vi "Overlays_test.vi"() -> ()   [LabVIEW 2018]
panel:
  out "Waveform Chart":cluster{dbl, dbl}(graph)
  in  "Stop":bool
  in  "Image Display":T1(plugin-control)
  out "size(s)":i32[](array[numeric])
  in  "Overlay Object":path=path "D:/Users_Data/Dmitriy_T/Documents/Tracker/TestVI's/Overlay_Object.png"
  in  "Overlay Bgr":path=path "D:/Users_Data/Dmitriy_T/Documents/Tracker/TestVI's/Overlay_Bgr.png"
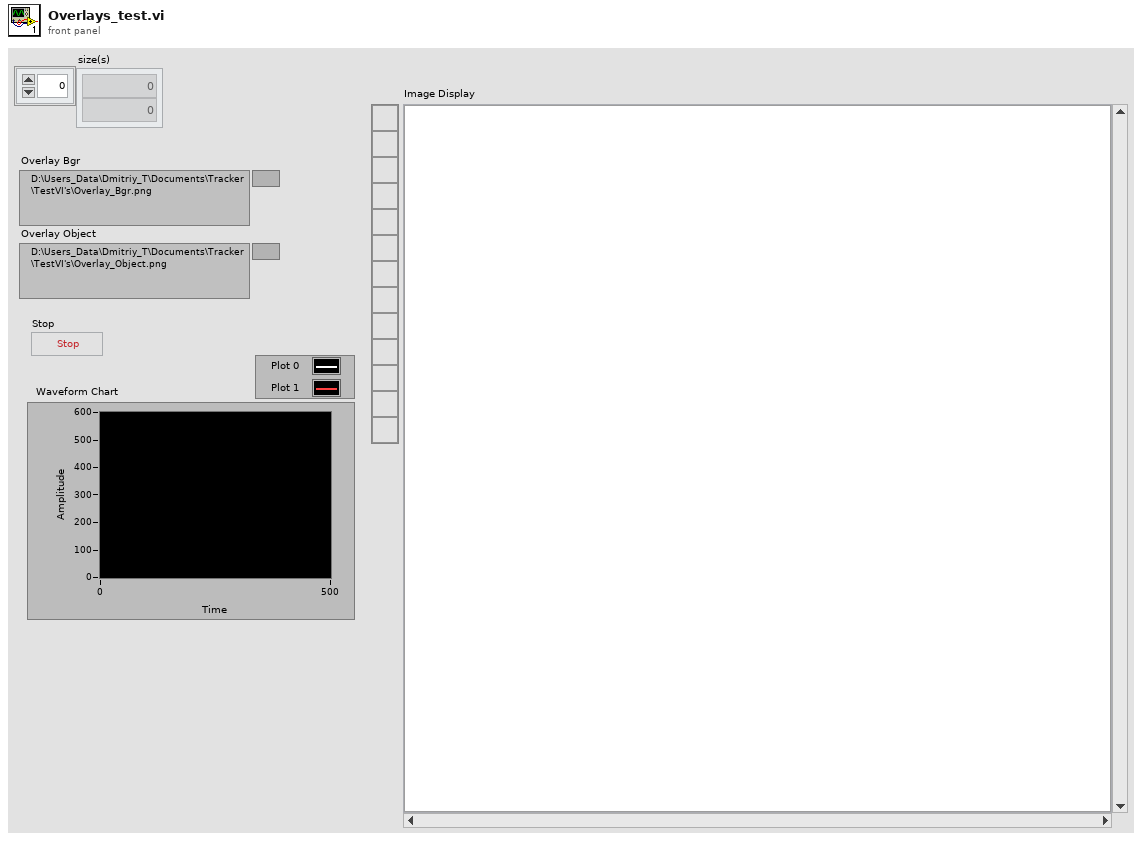
[diagram p1: front panel]
types:
  T1 = typedef "IMAQ Image.ctl" = refnum<image>
  T2 = typedef "Image Type" = u32
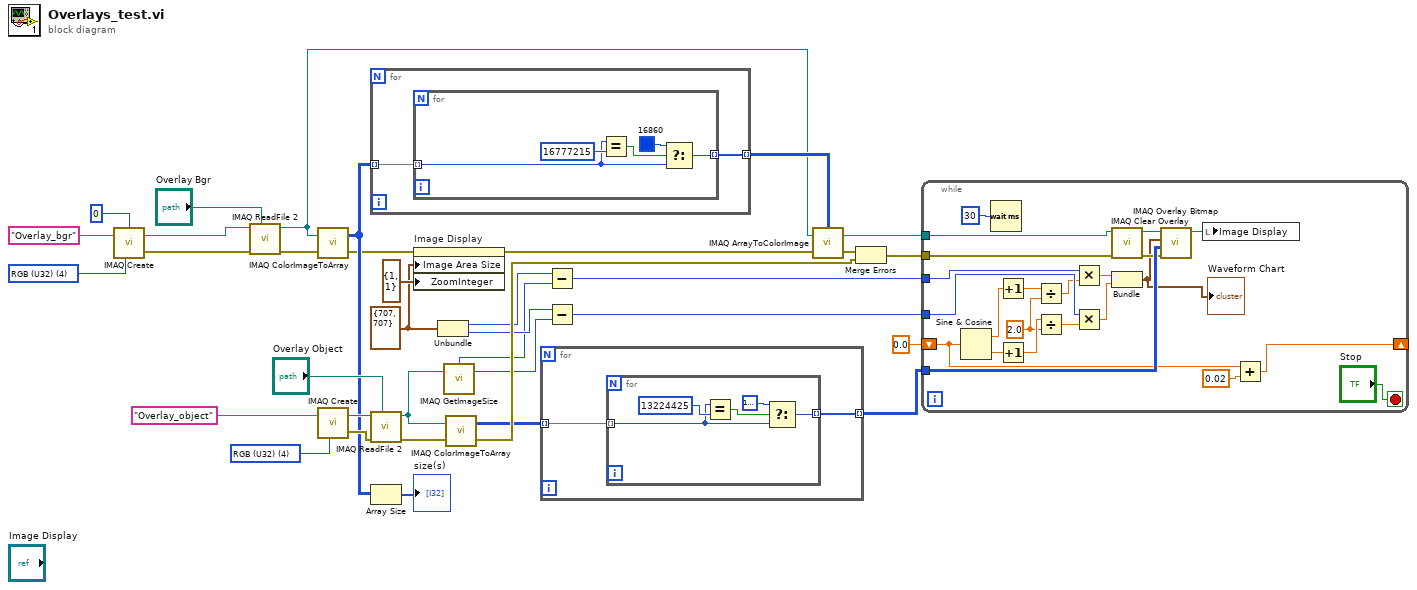
[diagram p0: block diagram]
diagram:
  w10 = cluster{"Width":u32, "Height":u32} {"Width"=707, "Height"=707} ("Image Area:Size:All Elements")
  w33 = T2 4 items=["Grayscale (U8)", "Grayscale (I16)", "Grayscale (SGL)", "Complex (CSG)", "RGB (U32)", "HSL (U32)", "RGB (U64)", "Grayscale (U16)"] ("Image Type")
  w34 = T2 4 items=["Grayscale (U8)", "Grayscale (I16)", "Grayscale (SGL)", "Complex (CSG)", "RGB (U32)", "HSL (U32)", "RGB (U64)", "Grayscale (U16)"] ("Image Type")
  n1 = call "IMAQ Create"("Border Size"=0, "Image Name"="Overlay_bgr", "Image Type"=w34) -> ("New Image"=w31:T1, "error out"=w29:errorcluster)  [unwired: 2 in]
  n2 = call "IMAQ ReadFile 2"("File Path"="Overlay Bgr", "error in (no error)"=w29, "Image"=w31) -> ("error out"=w21:errorcluster, "Image Out"=w18:T1)  [unwired: 4 in, 3 out]
  n3 = call "IMAQ ColorImageToArray"("Image"=w18, "error in (no error)"=w21) -> ("Image Pixels (U32)"=w17:u32[][], "error out"=w15:errorcluster)  [unwired: 2 in, 1 out]
  n4 = call "IMAQ Create"("Image Name"="Overlay_object", "Image Type"=w33) -> ("New Image"=w28:T1, "error out"=w27:errorcluster)  [unwired: 3 in]
  n5 = for {
    tunnel: w17 -> [w37] mode=indexing
    tunnel: [w36] -> w22 mode=indexing
    n6 = for {
      tunnel: w37 -> [w39] mode=indexing
      tunnel: [w41] -> w36 mode=indexing
      n7 = Equal?(x=w39, y=u32 16777215) -> (x = y?=w40:bool)
      n8 = Select(t=u32 16860, s=w40, f=w39) -> (s? t:f=w41:u32)
    }
  }
  n9 = call "IMAQ ReadFile 2"("File Path"="Overlay Object", "error in (no error)"=w27, "Image"=w28) -> ("error out"=w25:errorcluster, "Image Out"=w7:T1)  [unwired: 4 in, 3 out]
  n10 = Array Size(array=w17) -> (size(s)=→"size(s)":i32[])
  n11 = property on="Image Display" class="ImageControl"(error in=w15, "Image Area Size"=w10, "ZoomInteger"=cluster{"X":i32, "Y":i32} {"X"=1, "Y"=1} ("ZoomInteger:All Elements")) -> (error out=w14:errorcluster)  [unwired: 1 in, 1 out]
  n12 = Unbundle(w10) -> ("Width"=w9:u32, "Height"=w8:u32)
  n13 = call "IMAQ GetImageSize"("Image"=w7) -> ("Y Resolution"=w3:i32, "X Resolution"=w5:i32)  [unwired: 3 in, 1 out]
  n14 = call "IMAQ ColorImageToArray"("Image"=w7, "error in (no error)"=w25) -> ("Image Pixels (U32)"=w2:u32[][], "error out"=w24:errorcluster)  [unwired: 2 in, 1 out]
  n15 = for {
    tunnel: w2 -> [w44] mode=indexing
    tunnel: [w43] -> w1 mode=indexing
    n16 = for {
      tunnel: w44 -> [w46] mode=indexing
      tunnel: [w48] -> w43 mode=indexing
      n17 = Equal?(x=w46, y=u32 13224425) -> (x = y?=w47:bool)
      n18 = Select(t=u32 16777216, s=w47, f=w46) -> (s? t:f=w48:u32)
    }
  }
  n19 = Subtract(x=w9, y=w5) -> (x-y=w6:u32)
  n20 = Subtract(x=w8, y=w3) -> (x-y=w4:u32)
  n21 = call "IMAQ ArrayToColorImage"("Image Pixels (U32)"=w22, "Image"=w18, "error in (no error)"=w14) -> ("Image Out"=w19:T1, "error out"=w20:errorcluster)  [unwired: 2 in]
  n22 = Merge Errors(w20, w24) -> (w23:errorcluster)
  n23 = while {
    tunnel: w1 -> [w72]
    tunnel: w23 -> [w52]
    tunnel: w19 -> [w71]
    shift-right: [w67] -> _
    shift-left: 0.0 -> [w69]
    tunnel: w6 -> [w66]
    tunnel: w4 -> [w64]
    stop <- "Stop" stop-if-true
    w55 = 2.0 ("y")
    n24 = Sine & Cosine(0:w69) -> (1:w65:dbl, 2:w63:dbl)
    n25 = Wait (ms)(milliseconds to wait=u32 30) -> ()  [unwired: 1 out]
    n26 = Increment(x=w65) -> (x+1=w59:dbl)
    n27 = Increment(x=w63) -> (x+1=w58:dbl)
    n28 = Divide(x=w59, y=w55) -> (x/y=w57:dbl)
    n29 = Divide(x=w58, y=w55) -> (x/y=w56:dbl)
    n30 = Multiply(x=w66, y=w57) -> (x*y=w61:dbl)
    n31 = Multiply(x=w64, y=w56) -> (x*y=w62:dbl)
    n32 = call "IMAQ Clear Overlay"("error in (no error)"=w52, "Image"=w71) -> ("error out"=w51:errorcluster, "Image Out"=w53:T1)  [unwired: 8 in]
    n33 = Bundle(w61, w62) -> (w50:cluster{dbl, dbl})  [unwired: 1 in]
    "Waveform Chart" <- w50
    n34 = call "IMAQ Overlay Bitmap"("error in (no error)"=w51, "Bitmap"=w72, "Top Left Point"=w50, "Image"=w53) -> ("Image Out"=w54:T1)  [unwired: 6 in, 1 out]
    n35 = local write "Image Display"(w54) -> ()
    n36 = Add(x=w69, y=0.02) -> (x+y=w67:dbl)
  }
